vi "Store Tovey Data.vi"(8 "error in (no error)":errorcluster, 11 "Model in":refnum<class "Model.lvclass">) -> (0 "error out":errorcluster, 3 "Model out":refnum<class "Model.lvclass">)   [LabVIEW 2015, in "Model.lvclass"]
uses:
  Model.lvclass
  Model.lvclass/Model.ctl
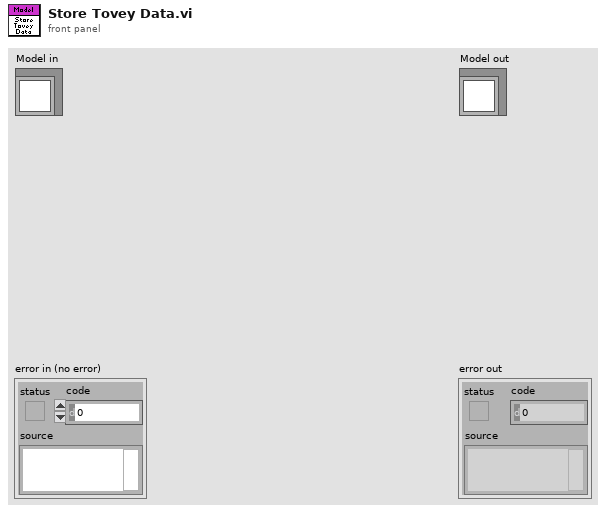
[diagram p1: front panel]
types:
  T1 = typedef "FAMT Typedefs.lvlib/ToveyEngData.ctl" = cluster{"Timestamp":dbl, "Fx":dbl, "Fy":dbl, "Fz":dbl, "Mx":dbl, "My":dbl, "Mz":dbl}
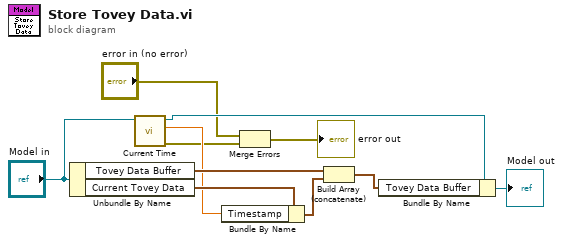
[diagram p0: block diagram]
diagram:
  n1 = Unbundle By Name("Model in") -> ("Tovey Data Buffer"=w11:T1[], "Current Tovey Data"=w8:T1)
  n2 = call "Current Time.vi"("Model in"="Model in") -> ("error out"=w3:errorcluster, "Time"=w4:dbl, "Model out"=w5:refnum<class "Model.lvclass">)  [unwired: 8 in]
  n3 = Bundle By Name(cluster=w8, "Timestamp"=w4) -> (w7:T1)
  n4 = Merge Errors("error in (no error)", w3) -> (→"error out":errorcluster)
  n5 = Build Array (concatenate)(w11, w7) -> (w10:T1[])
  n6 = Bundle By Name(cluster=w5, "Tovey Data Buffer"=w10) -> (→"Model out":refnum<class "Model.lvclass">)
